vi "niRFUtil MASMT RMS (CSG).vi"(8 "error in (no error)":errorcluster, 11 "X":csg[](array[numeric])) -> (0 "error out":errorcluster, 3 "rms":sgl)   [LabVIEW 2015, in "niRFUtil.lvlib"]
doc: "Computes the root mean square (rms) of the input sequence <B>X</B>."
uses:
  niRFUtil.lvlib
  Utilities/niRFMASMT_LINALG.dll
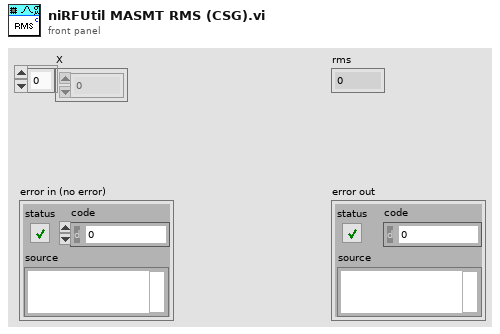
[diagram p1: front panel]
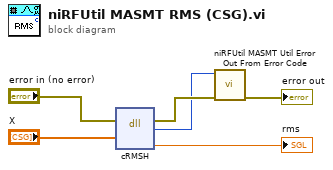
[diagram p0: block diagram]
diagram:
  n1 = dll-call lib="C:/Perforce/semoore-sales/Customers/NATI-3813/Noise Floor/LV Filters/ParallelComplexFilterRFUtil/niRFUtil/MASMT/Utilities/niRFMASMT_LINALG.*" fn="cRMSH"(error in="error in (no error)", "aH"="X") -> (error out=w3:errorcluster, "return type"=w2:i32, "rms"=→"rms":sgl)  [unwired: 4 in, 1 out]
  n2 = call "niRFUtil MASMT Util Error Out From Error Code.vi"("error in (no error)"=w3, "error code"=w2) -> ("error out"=→"error out":errorcluster)  [unwired: 9 in]
